vi "Flatten Data and Write to XML File.vi"() -> ()   [LabVIEW 2023]
doc: "Generates and displays an array of data, and calculates the max, min, and average values. The VI then flattens this data to XML and writes it to a file."
uses:
  support/Random Graph Data.ctl
  <vilib>/Analysis/baseanly.llb/Mean (DBL).vi
  <vilib>/Utility/xml.llb/Write to XML File.vi
  <vilib>/Analysis/NI_AALBase.lvlib
panel:
  out "Generated XML":string
  out "Graph":T1(graph)
  out "Max":dbl
  out "Min":dbl
  out "Mean":dbl
  # "Overview: Demonstrates the use of the LabVIEW Schema VIs and functions to flatten data and write it to an XML file that follows the LabVIEW-specific schema.\nInstructions:\n1. Run this VI.\n2. Open Read from XML File and Unflatten Data.vi and follow the instructions on its front panel."
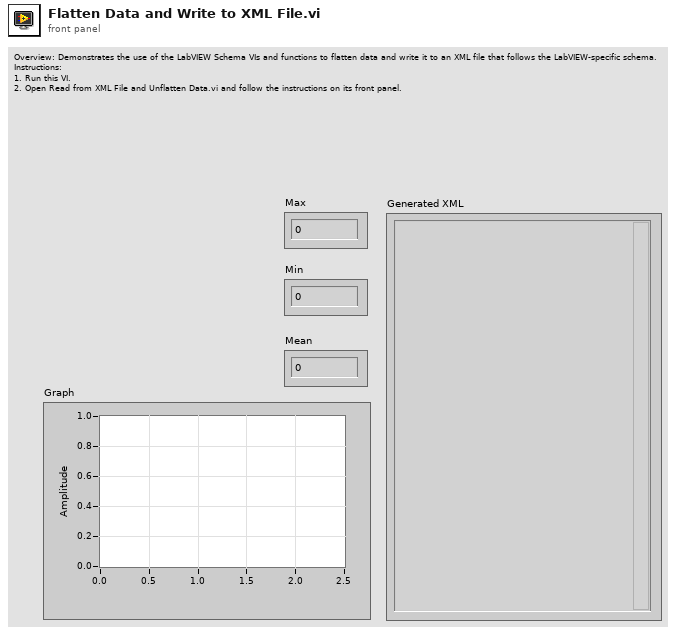
[diagram p1: front panel]
types:
  T1 = cluster{"Initial X":dbl, "Delta X":dbl, "Values":dbl[]}
  T2 = typedef "Random Graph Data.ctl" = cluster{"Initial X":dbl, "Delta X":dbl, "Values":dbl[]}
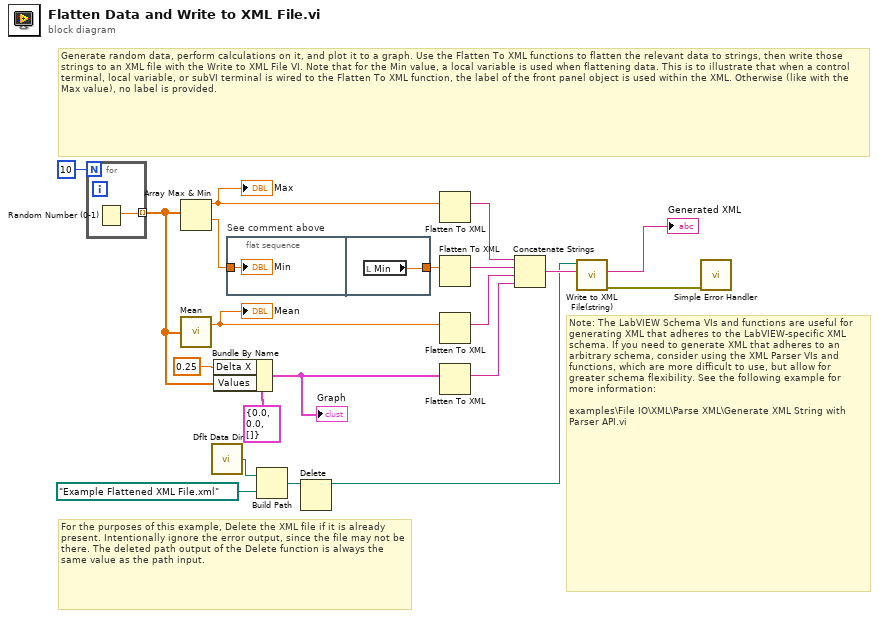
[diagram p0: block diagram]
diagram:
  # "Note: The LabVIEW Schema VIs and functions are useful for generating XML that adheres to the LabVIEW-specific XML schema. If you need to generate XML that adheres to an arbitrary schema, consider using the XML Parser VIs and functions, which are more difficult to use, but allow for greater schema flexibility. See the following example for more information:\n\nexamples\\File IO\\XML\\Parse XML\\Generate XML String with Parser API.vi"
  # "Generate random data, perform calculations on it, and plot it to a graph. Use the Flatten To XML functions to flatten the relevant data to strings, then write those strings to an XML file with the Write to XML File VI. Note that for the Min value, a local variable is used when flattening data. This is to illustrate that when a control terminal, local variable, or subVI terminal is wired to the Flatten To XML function, the label of the front panel object is used within the XML. Otherwise (like with the Max value), no label is provided."
  # "For the purposes of this example, Delete the XML file if it is already present. Intentionally ignore the error output, since the file may not be there. The deleted path output of the Delete function is always the same value as the path input."
  n1 = for {
    N: 10 -> [_]
    tunnel: [w21] -> w20 mode=indexing
    n2 = Random Number (0-1)() -> (number: 0 to 1=w21:dbl)
  }
  n3 = Array Max & Min ("Max & Min")(array=w20) -> (max value=w19:dbl, min value=w12:dbl)  [unwired: 2 out]
  "Max" <- w19
  n4 = call-poly <vilib>:"Mean.vi"("X"=w20) -> ("mean"=w18:dbl)  [unwired: 1 out]
  "Mean" <- w18
  n5 = call <vilib>:"Dflt Data Dir.vi"() -> ("App:Default Data Directory"=w4:path)
  n6 = Bundle By Name(cluster=T2 {"Initial X"=0.0, "Delta X"=0.0, "Values"=[]} ("Random Graph Data"), "Delta X"=0.25, "Values"=w20) -> (w17:T2)
  "Graph" <- w17
  n7 = flat-sequence "See comment above" {
    tunnel: w12 -> [w22]
    tunnel: [w23] -> w9
    frame #0 {
      "Min" <- w22
    }
    frame #1 {
      n8 = local read "Min"() -> (w23:dbl)
    }
  }
  n9 = Build Path(base path=w4, name or relative path=path "Example Flattened XML File.xml" ("default name")) -> (appended path=w5:path)
  n10 = Delete(path (use dialog)=w5) -> (deleted path=w2:path)  [unwired: 4 in, 2 out]
  n11 = Flatten To XML(6:w19) -> (2:w16:string)
  n12 = Flatten To XML(6:w9) -> (2:w14:string)
  n13 = Flatten To XML(6:w18) -> (2:w13:string)
  n14 = Flatten To XML(6:w17) -> (2:w15:string)
  n15 = Concatenate Strings(w16, w14, w13, w15) -> (w11:string)
  n16 = call-poly <vilib>:"Write to XML File(string).vi"("XML Input"=w11, "XML File Path"=w2) -> ("error out"=w8:errorcluster, "XML String"=→"Generated XML":string)  [unwired: 3 in, 5 out]
  n17 = call <vilib>:"Simple Error Handler.vi"("error in (no error)"=w8) -> ()  [unwired: 1 in, 8 out]
